vi "format_parameters.vi"(11 "T1_parameters":T1) -> (2 "parameters_dbl":dbl[](array[numeric]), 3 "parameters_strg":string[](array[string]))   [LabVIEW 2014]
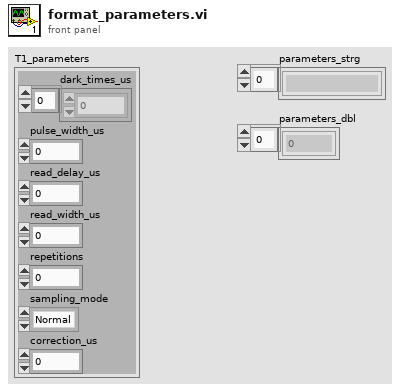
[diagram p1: front panel]
types:
  T1 = cluster{"dark_times_us":dbl[], "pulse_width_us":dbl, "read_delay_us":dbl, "read_width_us":dbl, "repetitions":i32, "sampling_mode":enum16{"Normal", "Sweep"}, "correction_us":dbl}
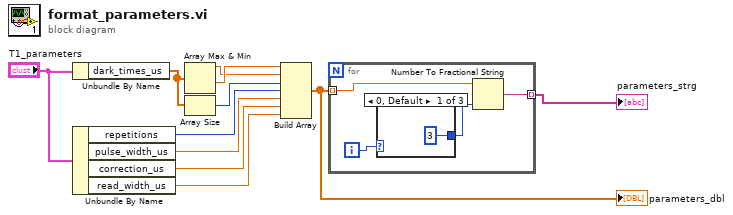
[diagram p0: block diagram]
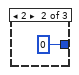
[diagram p2: hidden frame]
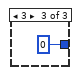
[diagram p3: hidden frame]
diagram:
  n1 = Unbundle By Name("T1_parameters") -> ("dark_times_us"=w11:dbl[])
  n2 = Unbundle By Name("T1_parameters") -> ("repetitions"=w6:i32, "pulse_width_us"=w5:dbl, "correction_us"=w4:dbl, "read_width_us"=w3:dbl)
  n3 = Array Max & Min(array=w11) -> (max value=w8:dbl, min value=w9:dbl)  [unwired: 2 out]
  n4 = Array Size(array=w11) -> (size(s)=w7:i32)
  n5 = Build Array(w9, w8, w7, w6, w5, w4, w3) -> (w2:dbl[])
  "parameters_dbl" <- w2
  n6 = for {
    tunnel: w2 -> [w14] mode=indexing
    tunnel: [w12] -> w1 mode=indexing
    i -> [w15]
    n7 = case shown="0, Default" w15 {
      tunnel: [i16 3 ("precision (6)") i16 0 ("precision (6)") i16 0 ("precision (6)")] -> w13
      frame 0, Default {
      }
      frame 2 {
      }
      frame 3 {
      }
    }
    n8 = Number To Fractional String(number=w14, precision (6)=w13) -> (F-format string=w12:string)  [unwired: 2 in]
  }
  "parameters_strg" <- w1
